vi "getState.vi"(8 "error in (no error)":errorcluster, 10 "index":i32, 11 "Channel.lvclass in":refnum<class "Channel.lvclass">) -> (0 "error out":errorcluster, 2 "state":cluster{"state_name":string, "value":string}, 3 "Channel.lvclass out":refnum<class "Channel.lvclass">)   [LabVIEW 2009, in "Tools.lvlib" / "DatabaseHelpers.lvlib" / "Channel.lvclass"]
uses:
  Channel.lvclass
  Channel.lvclass/Channel.ctl
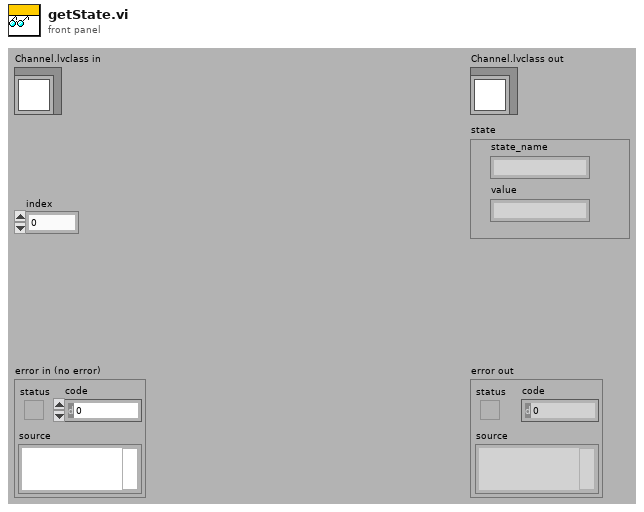
[diagram p1: front panel]
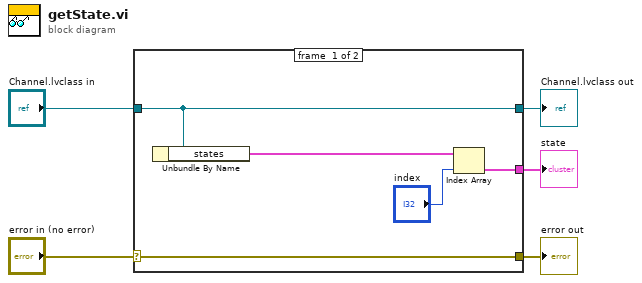
[diagram p0: block diagram]
diagram:
  n1 = case shown="No Error" "error in (no error)" {
    selector: "error in (no error)" -> [w10 w11]
    tunnel: [w10 w11] -> w4
    tunnel: [w9 w12] -> w2
    tunnel: "Channel.lvclass in" -> [w9 w12]
    tunnel: [w6 _] -> w1
    frame #0 {
      n2 = Unbundle By Name(w9) -> ("states"=w8:cluster{"state_name":string, "value":string}[])
      n3 = Index Array(array=w8, index="index") -> (element=w6:cluster{"state_name":string, "value":string})
    }
    frame #1 {
    }
  }
  "error out" <- w4
  "Channel.lvclass out" <- w2
  "state" <- w1
